vi "TranslateModbusInput.vi"(11 "ModbusInput":u16) -> (2 "ASCII Number Output":u8, 3 "Is Data?":bool)   [LabVIEW 2016, in "FPGAMockGyro.lvlib"]
uses:
  FPGAMockGyro.lvlib
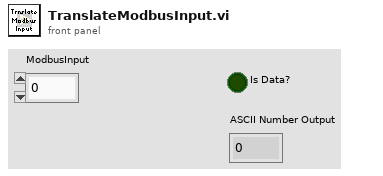
[diagram p1: front panel]
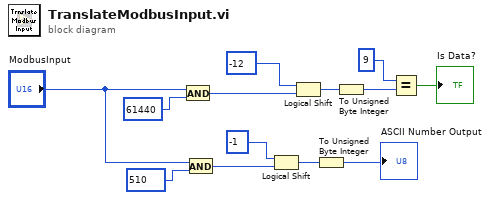
[diagram p0: block diagram]
diagram:
  n1 = And(x="ModbusInput", y=u16 61440) -> (x .and. y?=w10:u16)
  n2 = And(x="ModbusInput", y=u16 510) -> (x .and. y?=w7:u16)
  n3 = Logical Shift(y=i16 -1, x=w7) -> (x << y=w12:u16)
  n4 = Logical Shift(y=i16 -12, x=w10) -> (x << y=w13:u16)
  n5 = To Unsigned Byte Integer(number=w12) -> (unsigned 8bit integer=→"ASCII Number Output":u8)
  n6 = To Unsigned Byte Integer(number=w13) -> (unsigned 8bit integer=w4:u8)
  n7 = Equal?(x=u8 9, y=w4) -> (x = y?=→"Is Data?":bool)
